vi "Begin.vi"(8 "error in":errorcluster) -> (0 "error out":errorcluster)   [LabVIEW 2016]
doc: "Called before other user functions, this VI is expected to open initial I/O refnums, load in file data, and do all program initialization. Notice that the <B>error out</B> terminal is simply used for data flow. Wiring it to other structures or subVIs ensures that this VI runs first."
uses:
  <vilib>/Rock Robotics/WPI/DriverStation/WPI_DriverStationRobotMode2.ctl
  <vilib>/Rock Robotics/WPI/Joystick/WPI_JoystickDeviceEnum.ctl
  <vilib>/Rock Robotics/WPI/ThirdParty/CanMotor/TalonSRX/WPI_CANTalonSRX_APIControlMode.ctl
  <vilib>/Rock Robotics/WPI/ThirdParty/CanMotor/TalonSRX/WPI_CANTalonSRX_APIFeedbackSelect.ctl
  <vilib>/Rock Robotics/SystemInterfaces/DIO/FPGA_DIOPWMChannel.ctl
  <vilib>/Rock Robotics/SystemInterfaces/DIO/FPGA_DIOChannel.ctl
  Robot Global Data.vi
  <vilib>/Rock Robotics/Network Tables/NT Write String Array.vi
  <vilib>/Rock Robotics/WPI/MotorControl/WPI_MotorControlOpen VictorSP.vi
  <vilib>/Rock Robotics/WPI/ThirdParty/Sensors/Pigeon IMU/CTRE_PigeonIMU_Open_CAN.vi
  <vilib>/Rock Robotics/WPI/ThirdParty/Sensors/Pigeon IMU/CTRE_PigeonIMU_Open_TalonSRX.vi
  <vilib>/Rock Robotics/SystemInterfaces/AI/FPGA_AIChannel.ctl
panel:
  in  "PIDF Shooter":T1
  in  "PIDF Right":T1
  in  "PIDF Left":T1
  in  "CompBot?":bool=TRUE
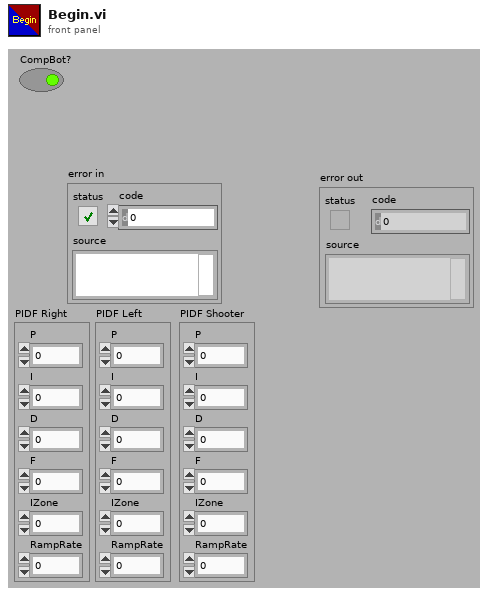
[diagram p1: front panel]
types:
  T1 = cluster{"P":dbl, "I":dbl, "D":dbl, "F":dbl, "IZone":dbl, "RampRate":dbl}
  T2 = typedef "FPGA_DIOChannel.ctl" = enum8{"DIO 0", "DIO 1", "DIO 2", "DIO 3", "DIO 4", "DIO 5", "DIO 6", "DIO 7", "DIO 8", "DIO 9", "DIO MXP 0", "DIO MXP 1", "DIO MXP 2", "DIO MXP 3", "DIO MXP 4", "DIO MXP 5", "DIO MXP 6", "DIO MXP 7", "DIO MXP 8", "DIO MXP 9", "DIO MXP 10", "DIO MXP 11", "DIO MXP 12", "DIO MXP 13", "DIO MXP 14", "DIO MXP 15", "SPI Port CS1", "SPI Port CS2", "SPI Port CS3", "SPI Port MISO", "SPI Port MOSI", "Invalid"}
  T3 = typedef "FPGA_DIOPWMChannel.ctl" = enum8{"PWM 0", "PWM 1", "PWM 2", "PWM 3", "PWM 4", "PWM 5", "PWM 6", "PWM 7", "PWM 8", "PWM 9", "PWM MXP 0", "PWM MXP 1", "PWM MXP 2", "PWM MXP 3", "PWM MXP 4", "PWM MXP 5", "PWM MXP 6", "PWM MXP 7", "PWM MXP 8", "PWM MXP 9", "Invalid"}
  T4 = typedef "WPI_CANTalonSRX_APIControlMode.ctl" = enum8{"Percent VBus", "Speed", "Position", "Slave", "Unchanged / Invalid", "Voltage Compensation", "Current", "Motion Profile", "Motion Magic"}
  T5 = typedef "WPI_CANTalonSRX_APIFeedbackSelect.ctl" = enum16{"Digital Quadrature Encoder", "Analog Potentiometer", "Analog Encoder", "Count on Quad-A (Rising-Edge)", "Count on Quad-A (Falling-Edge)", "CTR Magnetic Enc (Absolute)", "CTR Magnetic Enc (Relative)", "Pulse Width"}
  T6 = typedef "WPI_JoystickDeviceEnum.ctl" = enum16{"USB 0", "USB 1", "USB 2", "USB 3", "USB 4", "USB 5"}
  T7 = typedef "WPI_DriverStationRobotMode2.ctl" = enum16{"Autonomous Disabled", "Autonomous Enabled", "Teleop Disabled", "Teleop Enabled", "Disconnected", "Finish", "Test Disabled", "Test Enabled", "Emergency Stopped"}
  T8 = typedef "WPI_JoystickDevRef.ctl" = cluster{"Device":T6}
  T9 = typedef "WPI_MotorControlDeviceRef.ctl" = cluster{"DeviceStatus":errorcluster, "Type":T10, "PWM":cluster{"PWM Channel":T3, "DeadBand":T11}, "CAN":cluster{"Device Number":u8, "SetOutput VI Ref":variant, "GetOutput VI Ref":variant, "Enable VI Ref":variant, "Disable VI Ref":variant, "Data":variant}, "Invert":bool}
  T10 = typedef "WPI_MotorControlType.ctl" = enum16{"PWM", "CAN"}
  T11 = typedef "WPI_PWMDeadband.ctl" = cluster{"Name":string, "maxPositivePwm":i32, "minPositivePwm":i32, "centerPwm":i32, "maxNegativePwm":i32, "minNegativePwm":i32, "angularRange":u16}
  T12 = typedef "CTRE_PigeonIMU_DeviceRef.ctl" = cluster{"DeviceStatus":errorcluster, "Device Number":u8, "Type":T13, "Device ID":u32}
  T13 = typedef "CTRE_PigeonIMU_ConnectionType.ctl" = u32
  T14 = typedef "FPGA_AIChannel.ctl" = enum8{"AI 0", "AI 1", "AI 2", "AI 3", "AI MXP 0", "AI MXP 1", "AI MXP 2", "AI MXP 3", "Invalid"}
  T15 = typedef "WPI_PotentiometerDevRef.ctl" = cluster{"DevStatus":errorcluster, "Analog Channel":T14, "Invert Output":bool}
  T16 = typedef "WPI_DriverStationAllianceInfo.ctl" = enum16{"Red", "Blue", "Invalid"}
  T17 = typedef "WPI_DigitalInputDevRef.ctl" = cluster{"DevStatus":errorcluster, "DIO Channel":T2}
  T18 = enum16{"OFF", "RED", "GREEN", "BLUE", "PURPLE", "YELLOW", "TEAL", "WHITE", "RAINBOW"}
  T19 = typedef "WPI_ServoDeviceRef.ctl" = cluster{"DeviceStatus":errorcluster, "PWM Channel":T3, "DeadBand":T11}
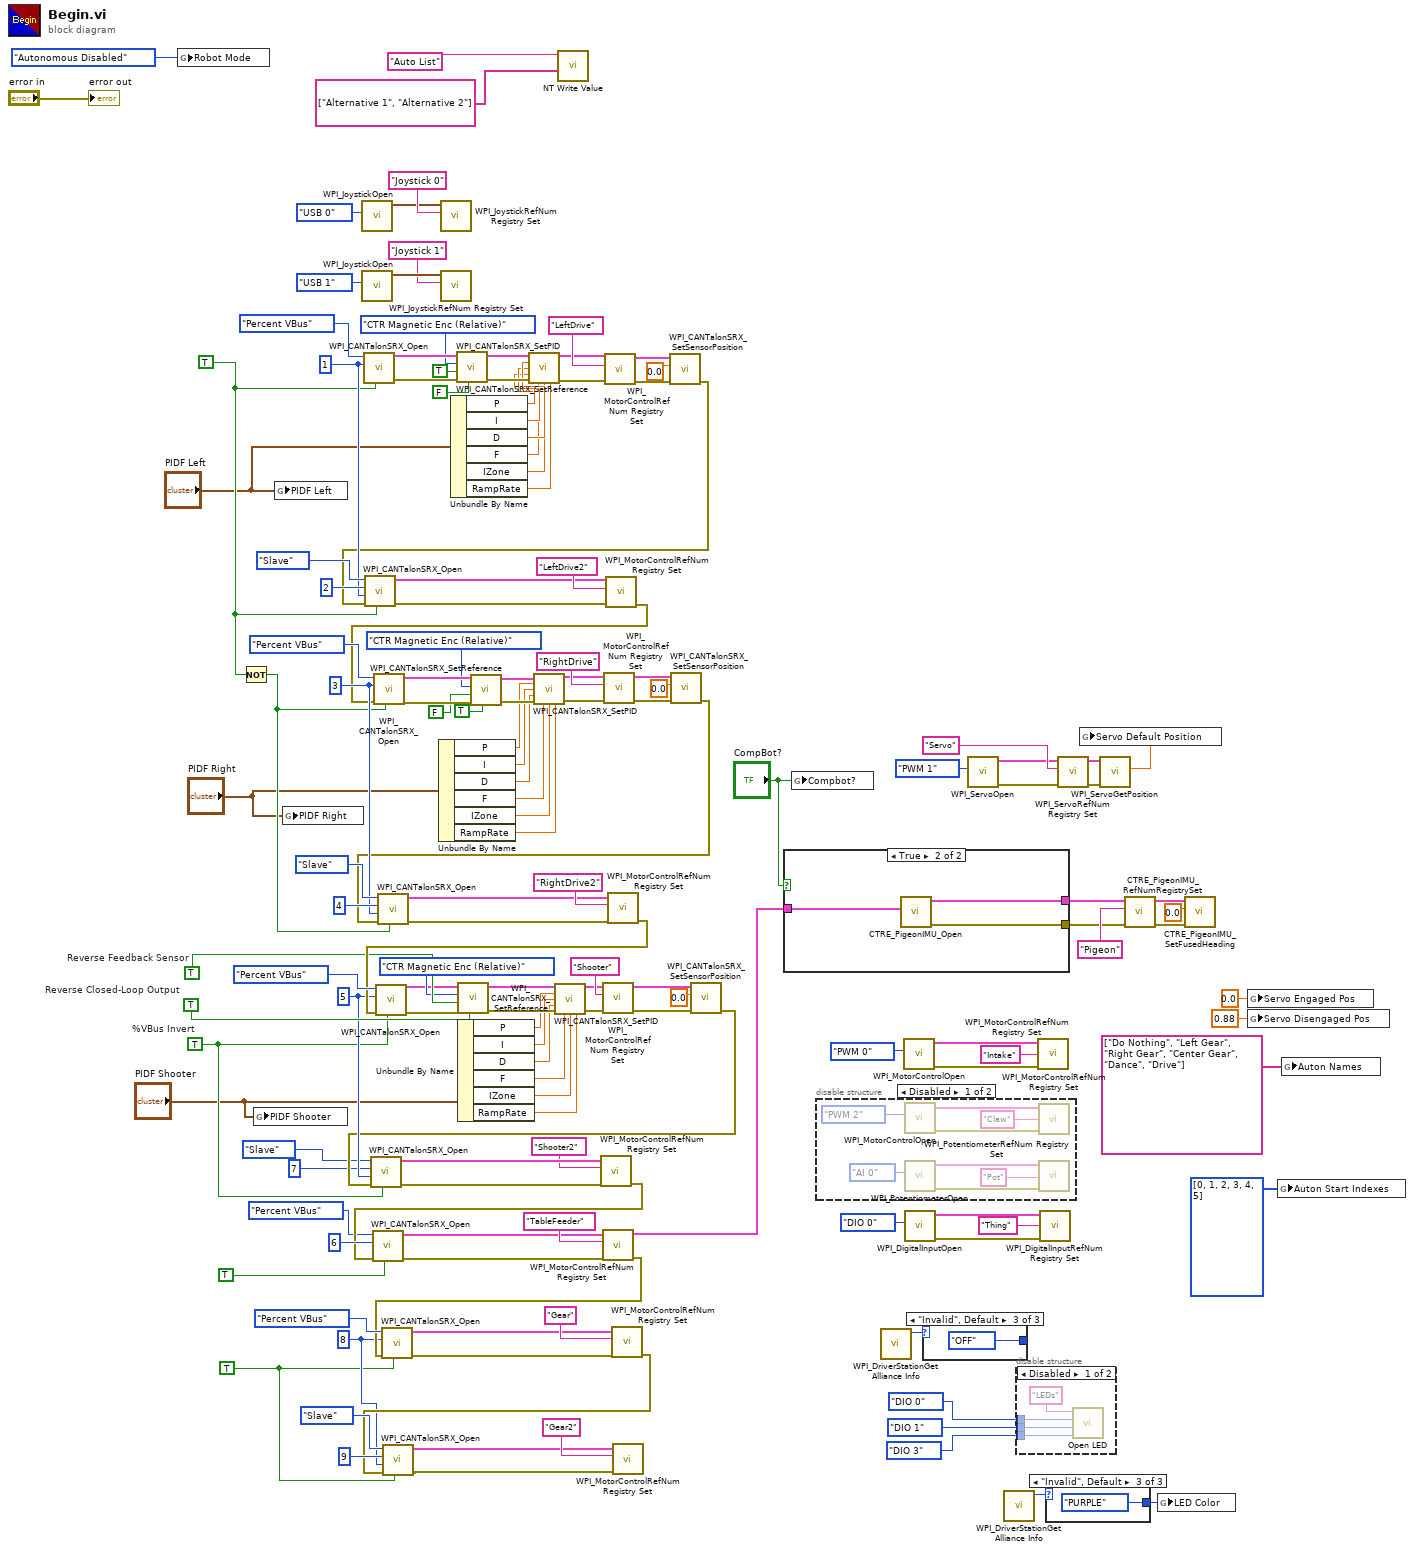
[diagram p0: block diagram]
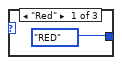
[diagram p3: hidden frame]
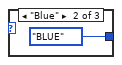
[diagram p4: hidden frame]
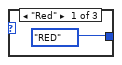
[diagram p5: hidden frame]
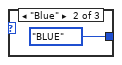
[diagram p6: hidden frame]
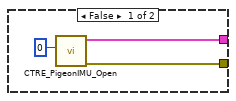
[diagram p8: hidden frame]
diagram:
  w79 = TRUE  # %VBus Invert
  w93 = TRUE
  w94 = u8 8 ("Device Number")
  w115 = TRUE  # Reverse Closed-Loop Output
  w114 = TRUE  # Reverse Feedback Sensor
  w80 = u8 5 ("Device Number")
  w129 = TRUE
  w130 = u8 3 ("Device Number")
  w131 = u8 1 ("Device Number")
  n1 = global write "Robot Global Data.vi" "Robot Mode"(WPI_DriverStationRobotMode2."Autonomous Disabled" ("Robot Mode")) -> ()
  n2 = Not(x=w129) -> (.not. x?=w128:bool)
  n3 = global write "Robot Global Data.vi" "PIDF Shooter"("PIDF Shooter") -> ()
  n4 = global write "Robot Global Data.vi" "PIDF Left"("PIDF Left") -> ()
  n5 = global write "Robot Global Data.vi" "PIDF Right"("PIDF Right") -> ()
  n6 = call <vilib>:"WPI_JoystickOpen.vi"("JoystickDevice"=WPI_JoystickDeviceEnum."USB 0") -> ("JoystickDevRef"=w149:T8)  [unwired: 10 in]
  n7 = call <vilib>:"WPI_JoystickOpen.vi"("JoystickDevice"=WPI_JoystickDeviceEnum."USB 1") -> ("JoystickDevRef"=w110:T8)  [unwired: 10 in]
  n8 = call <vilib>:"WPI_CANTalonSRX_Open.vi"("Invert"=w129, "Device Number"=w131, "Control Mode"=WPI_CANTalonSRX_APIControlMode."Percent VBus") -> ("error out"=w83:errorcluster, "CAN Talon SRX Ref"=w85:T9)  [unwired: 7 in]
  n9 = Unbundle By Name("PIDF Right") -> ("P"=w40:dbl, "I"=w39:dbl, "D"=w38:dbl, "F"=w37:dbl, "IZone"=w36:dbl, "RampRate"=w35:dbl)
  n10 = call <vilib>:"WPI_JoystickRefNum Registry Set.vi"("refnum name"="Joystick 0", "JoystickDevRef"=w149) -> ()  [unwired: 8 in, 2 out]
  n11 = call <vilib>:"WPI_JoystickRefNum Registry Set.vi"("refnum name"="Joystick 1", "JoystickDevRef"=w110) -> ()  [unwired: 8 in, 2 out]
  n12 = Unbundle By Name("PIDF Left") -> ("P"=w50:dbl, "I"=w49:dbl, "D"=w48:dbl, "F"=w47:dbl, "IZone"=w46:dbl, "RampRate"=w45:dbl)
  n13 = call <vilib>:"WPI_CANTalonSRX_SetReference.vi"("Reverse Closed-Loop Output"=FALSE, "error in (no error)"=w83, "Reverse Feedback Sensor"=TRUE, "Feedback Reference"=WPI_CANTalonSRX_APIFeedbackSelect."CTR Magnetic Enc (Relative)", "CAN Talon SRX Ref"=w85) -> ("error out"=w52:errorcluster, "CAN Talon SRX Ref"=w84:T9)  [unwired: 5 in]
  n14 = Unbundle By Name("PIDF Shooter") -> ("P"=w30:dbl, "I"=w29:dbl, "D"=w28:dbl, "F"=w27:dbl, "IZone"=w26:dbl, "RampRate"=w25:dbl)
  n15 = call <vilib>:"WPI_CANTalonSRX_SetPID.vi"("CAN Talon SRX Ref"=w84, "P"=w50, "I"=w49, "D"=w48, "error in (no error)"=w52, "F"=w47, "I Zone"=w46, "Ramp Rate"=w45) -> ("CAN Talon SRX Ref"=w53:T9, "error out"=w51:errorcluster)  [unwired: 6 in]
  n16 = call-poly <vilib>:"NT Write Value.vi"("String Array"=string[] ["Alternative 1", "Alternative 2"], "Name"="Auto List") -> ()  [unwired: 9 in, 1 out]
  n17 = call <vilib>:"WPI_MotorControlRefNum Registry Set.vi"("error in (no error)"=w51, "refnum name"="LeftDrive", "MotorControlDevRef"=w53) -> ("error out"=w70:errorcluster, "MotorControlDevRef"=w69:T9)  [unwired: 7 in]
  n18 = call <vilib>:"WPI_CANTalonSRX_SetSensorPosition.vi"("error in (no error)"=w70, "New Sensor Position"=0.0, "CAN Talon SRX Ref"=w69) -> ("error out"=w68:errorcluster)  [unwired: 7 in, 1 out]
  n19 = call <vilib>:"WPI_CANTalonSRX_Open.vi"("Invert"=w129, "error in"=w68, "Master Device Number"=w131, "Device Number"=u8 2, "Control Mode"=WPI_CANTalonSRX_APIControlMode."Slave") -> ("error out"=w138:errorcluster, "CAN Talon SRX Ref"=w139:T9)  [unwired: 5 in]
  n20 = call <vilib>:"WPI_MotorControlRefNum Registry Set.vi"("error in (no error)"=w138, "refnum name"="LeftDrive2", "MotorControlDevRef"=w139) -> ("error out"=w127:errorcluster)  [unwired: 7 in, 1 out]
  n21 = call <vilib>:"WPI_CANTalonSRX_Open.vi"("Invert"=w128, "error in"=w127, "Device Number"=w130, "Control Mode"=WPI_CANTalonSRX_APIControlMode."Percent VBus") -> ("error out"=w87:errorcluster, "CAN Talon SRX Ref"=w88:T9)  [unwired: 6 in]
  n22 = call <vilib>:"WPI_CANTalonSRX_SetReference.vi"("Reverse Closed-Loop Output"=TRUE, "error in (no error)"=w87, "Reverse Feedback Sensor"=FALSE ("Reverse Closed-Loop Output"), "Feedback Reference"=WPI_CANTalonSRX_APIFeedbackSelect."CTR Magnetic Enc (Relative)", "CAN Talon SRX Ref"=w88) -> ("error out"=w41:errorcluster, "CAN Talon SRX Ref"=w44:T9)  [unwired: 5 in]
  n23 = call <vilib>:"WPI_CANTalonSRX_SetPID.vi"("CAN Talon SRX Ref"=w44, "P"=w40, "I"=w39, "D"=w38, "error in (no error)"=w41, "F"=w37, "I Zone"=w36, "Ramp Rate"=w35) -> ("CAN Talon SRX Ref"=w43:T9, "error out"=w42:errorcluster)  [unwired: 6 in]
  n24 = call <vilib>:"WPI_MotorControlRefNum Registry Set.vi"("error in (no error)"=w42, "refnum name"="RightDrive", "MotorControlDevRef"=w43) -> ("error out"=w74:errorcluster, "MotorControlDevRef"=w73:T9)  [unwired: 7 in]
  n25 = call <vilib>:"WPI_CANTalonSRX_SetSensorPosition.vi"("error in (no error)"=w74, "New Sensor Position"=0.0, "CAN Talon SRX Ref"=w73) -> ("error out"=w72:errorcluster)  [unwired: 7 in, 1 out]
  n26 = call <vilib>:"WPI_CANTalonSRX_Open.vi"("Invert"=w128, "error in"=w72, "Master Device Number"=w130, "Device Number"=u8 4, "Control Mode"=WPI_CANTalonSRX_APIControlMode."Slave") -> ("error out"=w132:errorcluster, "CAN Talon SRX Ref"=w102:T9)  [unwired: 5 in]
  n27 = call <vilib>:"WPI_MotorControlRefNum Registry Set.vi"("error in (no error)"=w132, "refnum name"="RightDrive2", "MotorControlDevRef"=w102) -> ("error out"=w124:errorcluster)  [unwired: 7 in, 1 out]
  n28 = call <vilib>:"WPI_CANTalonSRX_Open.vi"("Invert"=w79, "error in"=w124, "Device Number"=w80, "Control Mode"=WPI_CANTalonSRX_APIControlMode."Percent VBus") -> ("error out"=w32:errorcluster, "CAN Talon SRX Ref"=w112:T9)  [unwired: 6 in]
  n29 = call <vilib>:"WPI_CANTalonSRX_SetReference.vi"("Reverse Closed-Loop Output"=w115, "Reverse Feedback Sensor"=w114, "Feedback Reference"=WPI_CANTalonSRX_APIFeedbackSelect."CTR Magnetic Enc (Relative)", "CAN Talon SRX Ref"=w112) -> ("CAN Talon SRX Ref"=w34:T9)  [unwired: 6 in, 1 out]
  n30 = call <vilib>:"WPI_CANTalonSRX_SetPID.vi"("CAN Talon SRX Ref"=w34, "P"=w30, "I"=w29, "D"=w28, "error in (no error)"=w32, "F"=w27, "I Zone"=w26, "Ramp Rate"=w25) -> ("CAN Talon SRX Ref"=w33:T9, "error out"=w31:errorcluster)  [unwired: 6 in]
  n31 = call <vilib>:"WPI_MotorControlRefNum Registry Set.vi"("error in (no error)"=w31, "refnum name"="Shooter", "MotorControlDevRef"=w33) -> ("error out"=w78:errorcluster, "MotorControlDevRef"=w77:T9)  [unwired: 7 in]
  n32 = call <vilib>:"WPI_CANTalonSRX_SetSensorPosition.vi"("error in (no error)"=w78, "New Sensor Position"=0.0, "CAN Talon SRX Ref"=w77) -> ("error out"=w76:errorcluster)  [unwired: 7 in, 1 out]
  n33 = call <vilib>:"WPI_CANTalonSRX_Open.vi"("Invert"=w79, "error in"=w76, "Master Device Number"=w80, "Device Number"=u8 7, "Control Mode"=WPI_CANTalonSRX_APIControlMode."Slave") -> ("error out"=w123:errorcluster, "CAN Talon SRX Ref"=w122:T9)  [unwired: 5 in]
  n34 = call <vilib>:"WPI_MotorControlRefNum Registry Set.vi"("error in (no error)"=w123, "refnum name"="Shooter2", "MotorControlDevRef"=w122) -> ("error out"=w117:errorcluster)  [unwired: 7 in, 1 out]
  n35 = call <vilib>:"WPI_CANTalonSRX_Open.vi"("Invert"=TRUE, "error in"=w117, "Device Number"=u8 6, "Control Mode"=WPI_CANTalonSRX_APIControlMode."Percent VBus") -> ("error out"=w118:errorcluster, "CAN Talon SRX Ref"=w119:T9)  [unwired: 6 in]
  n36 = call <vilib>:"WPI_MotorControlRefNum Registry Set.vi"("error in (no error)"=w118, "refnum name"="TableFeeder", "MotorControlDevRef"=w119) -> ("error out"=w96:errorcluster, "MotorControlDevRef"=w62:T9)  [unwired: 7 in]
  n37 = call <vilib>:"WPI_CANTalonSRX_Open.vi"("Invert"=w93, "error in"=w96, "Device Number"=w94, "Control Mode"=WPI_CANTalonSRX_APIControlMode."Percent VBus") -> ("error out"=w89:errorcluster, "CAN Talon SRX Ref"=w90:T9)  [unwired: 6 in]
  n38 = call <vilib>:"WPI_MotorControlRefNum Registry Set.vi"("error in (no error)"=w89, "refnum name"="Gear", "MotorControlDevRef"=w90) -> ("error out"=w95:errorcluster)  [unwired: 7 in, 1 out]
  n39 = call <vilib>:"WPI_CANTalonSRX_Open.vi"("Invert"=w93, "error in"=w95, "Master Device Number"=w94, "Device Number"=u8 9, "Control Mode"=WPI_CANTalonSRX_APIControlMode."Slave") -> ("error out"=w91:errorcluster, "CAN Talon SRX Ref"=w92:T9)  [unwired: 5 in]
  n40 = call <vilib>:"WPI_MotorControlRefNum Registry Set.vi"("error in (no error)"=w91, "refnum name"="Gear2", "MotorControlDevRef"=w92) -> ()  [unwired: 7 in, 2 out]
  n41 = case shown="True" "CompBot?" {
    tunnel: [w154 w156] -> w104
    tunnel: [w153 w157] -> w103
    tunnel: w62 -> [_ w155]
    frame False {
      n42 = call-poly <vilib>:"CTRE_PigeonIMU_Open.vi"("Device Number"=u8 0) -> ("error out"=w154:errorcluster, "PigeonIMUDevRef"=w153:T12)  [unwired: 9 in]
    }
    frame True {
      n43 = call-poly <vilib>:"CTRE_PigeonIMU_Open.vi"("CAN Talon SRX Ref"=w155) -> ("error out"=w156:errorcluster, "PigeonIMUDevRef"=w157:T12)  [unwired: 9 in]
    }
  }
  n44 = global write "Robot Global Data.vi" "Compbot?"("CompBot?") -> ()
  n45 = disable-structure shown="Disabled" {
    frame Disabled {
      n46 = call-poly <vilib>:"WPI_MotorControlOpen.vi"("PWM Channel"=FPGA_DIOPWMChannel."PWM 2") -> ("error out"=w163:errorcluster, "MotorControlDeviceRef"=w164:T9)  [unwired: 9 in]
      n47 = call <vilib>:"WPI_PotentiometerOpen.vi"("Analog Channel"=FPGA_AIChannel."AI 0") -> ("error out"=w161:errorcluster, "PotDevRef"=w160:T15)  [unwired: 9 in]
      n48 = call <vilib>:"WPI_MotorControlRefNum Registry Set.vi"("error in (no error)"=w163, "refnum name"="Claw", "MotorControlDevRef"=w164) -> ()  [unwired: 7 in, 2 out]
      n49 = call <vilib>:"WPI_PotentiometerRefNum Registry Set.vi"("error in (no error)"=w161, "refnum name"="Pot", "PotDevRef"=w160) -> ()  [unwired: 7 in, 2 out]
    }
    frame Enabled {
    }
  }
  n50 = call <vilib>:"WPI_DriverStationGet Alliance Info.vi"() -> ("Alliance"=w5:T16)  [unwired: 10 in, 1 out]
  n51 = call-poly <vilib>:"WPI_MotorControlOpen.vi"("PWM Channel"=FPGA_DIOPWMChannel."PWM 0") -> ("error out"=w61:errorcluster, "MotorControlDeviceRef"=w60:T9)  [unwired: 9 in]
  n52 = call <vilib>:"WPI_DigitalInputOpen.vi"("DIO Channel"=FPGA_DIOChannel."DIO 0") -> ("error out"=w23:errorcluster, "DigitalInputDevRef"=w24:T17)  [unwired: 9 in]
  n53 = case shown="\"Invalid\", Default" w5 {
    tunnel: [T18."RED" ("lower limit") T18."BLUE" ("lower limit") T18."OFF" ("lower limit")] -> _
    frame "Red" {
    }
    frame "Blue" {
    }
    frame "Invalid", Default {
    }
  }
  n54 = call <vilib>:"WPI_ServoOpen.vi"("PWM Channel"=FPGA_DIOPWMChannel."PWM 1") -> ("error out"=w13:errorcluster, "ServoDeviceRef"=w12:T19)  [unwired: 9 in]
  n55 = call <vilib>:"WPI_DriverStationGet Alliance Info.vi"() -> ("Alliance"=w4:T16)  [unwired: 10 in, 1 out]
  n56 = disable-structure shown="Disabled" {
    disable-tunnel: FPGA_DIOChannel."DIO 0" ("DIO Channel") -> [w172 _]
    disable-tunnel: FPGA_DIOChannel."DIO 1" ("DIO Channel") -> [w171 _]
    disable-tunnel: FPGA_DIOChannel."DIO 3" ("DIO Channel") -> [w170 _]
    frame Disabled {
      n57 = call "Open LED.vi"("DIO Channel Red"=w170, "DIO Channel Green"=w171, "DIO Channel Blue"=w172, "refnum name"="LEDs") -> ()  [unwired: 7 in, 1 out]
    }
    frame Enabled {
    }
  }
  n58 = call <vilib>:"WPI_MotorControlRefNum Registry Set.vi"("error in (no error)"=w61, "refnum name"="Intake", "MotorControlDevRef"=w60) -> ()  [unwired: 7 in, 2 out]
  n59 = call <vilib>:"WPI_DigitalInputRefNum Registry Set.vi"("error in (no error)"=w23, "refnum name"="Thing", "DigitalInputDevRef"=w24) -> ()  [unwired: 7 in, 2 out]
  n60 = case shown="\"Invalid\", Default" w4 {
    tunnel: [T18."RED" ("lower limit") T18."BLUE" ("lower limit") T18."PURPLE" ("lower limit")] -> w3
    frame "Red" {
    }
    frame "Blue" {
    }
    frame "Invalid", Default {
    }
  }
  n61 = call <vilib>:"WPI_ServoRefNum Registry Set.vi"("error in (no error)"=w13, "refnum name"="Servo", "ServoDeviceRef"=w12) -> ("error out"=w16:errorcluster, "ServoDeviceRef"=w17:T19)  [unwired: 7 in]
  n62 = call <vilib>:"WPI_ServoGetPosition.vi"("error in (no error)"=w16, "ServoDeviceRef"=w17) -> ("Position"=w11:dbl)  [unwired: 7 in, 2 out]
  n63 = global write "Robot Global Data.vi" "Servo Default Position"(w11) -> ()
  n64 = call <vilib>:"CTRE_PigeonIMU_RefNumRegistrySet.vi"("error in (no error)"=w104, "refnum name"="Pigeon", "PigeonIMUDevRef"=w103) -> ("error out"=w107:errorcluster, "PigeonIMUDevRef"=w106:T12)  [unwired: 7 in]
  n65 = global write "Robot Global Data.vi" "LED Color"(w3) -> ()
  n66 = call <vilib>:"CTRE_PigeonIMU_SetFusedHeading.vi"("error in (no error)"=w107, "Value"=0.0, "PigeonIMUDevRef 2"=w106) -> ()  [unwired: 7 in, 2 out]
  n67 = global write "Robot Global Data.vi" "Servo Engaged Pos"(0.0 ("Servo Engaged Pos")) -> ()
  n68 = global write "Robot Global Data.vi" "Servo Disengaged Pos"(0.88 ("Servo Disengaged Pos")) -> ()
  n69 = global write "Robot Global Data.vi" "Auton Start Indexes"(i32[] [0, 1, 2, 3, 4, 5] ("Auton Start Index")) -> ()
  n70 = global write "Robot Global Data.vi" "Auton Names"(string[] ["Do Nothing", "Left Gear", "Right Gear", "Center Gear", "Dance", "Drive"] ("Auton Name")) -> ()
  "error out" <- "error in"
